vi "get async cmd.vi"(10 "error in (no error)":errorcluster, 11 "Cmd String in":string) -> (2 "error out":errorcluster, 3 "AsyncCmd":T1)   [LabVIEW 2022 SP3, in "Database.lvclass"]
doc: "Developed by Kevin Thompson\nkevin@thompsonengineering.net\n\nCopyright 2018\nThompson Engineering, LLC"
uses:
  Database.lvclass
  DataTypes/AsynCmd_Temp01--enum.ctl
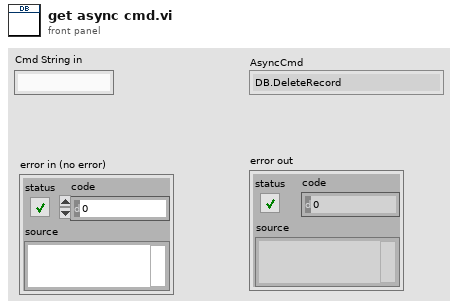
[diagram p1: front panel]
types:
  T1 = typedef "Database.lvclass/AsynCmd_Temp01--enum.ctl" = enum16{"DB.DeleteRecord", "DB.UpdateRecord", "DB.InsertRecord", "DB.SelectRecord", "DB.ExecuteSQLCommand", "DB.FindFirstSlot", "DB.GenericSQLQuery"}
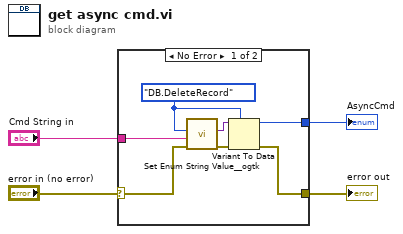
[diagram p0: block diagram]
diagram:
  n1 = case shown="No Error" "error in (no error)" {
    selector: "error in (no error)" -> [w5 w12]
    tunnel: "Cmd String in" -> [w10 _]
    tunnel: [w9 _] -> w3
    tunnel: [w6 w12] -> w2
    frame No Error {
      w8 = AsynCmd_Temp01--enum."DB.DeleteRecord" ("AsyncCmd")
      n2 = call <userlib>:"Set Enum String Value__ogtk.vi"("error in (no error)"=w5, "String Value"=w10, "Default Enum Value"=w8) -> ("error out"=w7:errorcluster, "Enum"=w11:variant)  [unwired: 7 in]
      n3 = Variant To Data(error in=w7, type=w8, Variant=w11) -> (data=w9:T1, error out=w6:errorcluster)
    }
    frame Error {
    }
  }
  "AsyncCmd" <- w3
  "error out" <- w2
